vi "Robo Team Send Pitch Rotation Command.vi"(7 "timeout in ms (5000)":i32=5000, 8 "error in (no error)":errorcluster, 10 "Data in":variant, 11 "Command":string) -> (0 "error out":errorcluster, 2 "Data out":variant)   [LabVIEW 2015]
uses:
  Robo Team Engine Command.ctl
  Robo Team Globals.vi
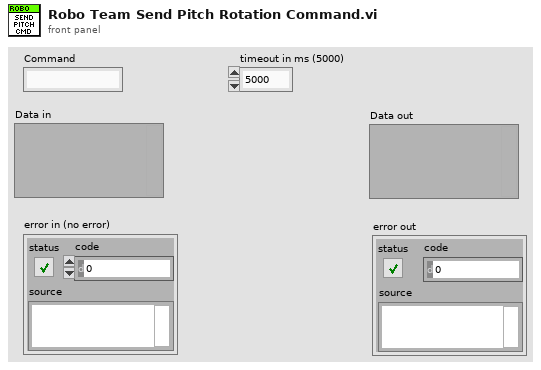
[diagram p1: front panel]
types:
  T1 = typedef "Robo Team Engine Command.ctl" = cluster{"Command":string, "Data":variant, "Error":errorcluster, "Timeout":i32}
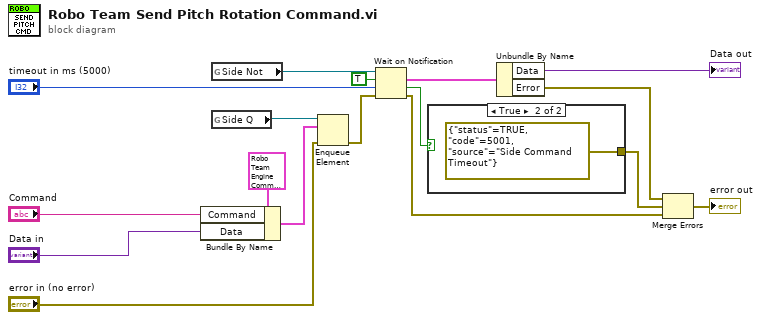
[diagram p0: block diagram]
diagram:
  n1 = Bundle By Name(cluster=T1 {"Command"="", "Data"=variant, "Error"={"status"=FALSE, "code"=0, "source"=""}, "Timeout"=0} ("element"), "Command"="Command", "Data"="Data in") -> (w12:T1)
  n2 = global read "Robo Team Globals.vi" "Side Not"() -> (w8:refnum<notifier>)
  n3 = global read "Robo Team Globals.vi" "Side Q"() -> (w7:refnum<queue>)
  n4 = Enqueue Element(queue=w7, element=w12, error in (no error)="error in (no error)") -> (error out=w9:errorcluster)  [unwired: 1 in, 2 out]
  n5 = Wait on Notification(notifier=w8, ignore previous (F)=TRUE, timeout in ms (-1)="timeout in ms (5000)", error in (no error)=w9) -> (notification=w14:T1, timed out?=w3:bool, error out=w5:errorcluster)  [unwired: 1 out]
  n6 = case shown="True" w3 {
    tunnel: [_ errorcluster {"status"=TRUE, "code"=5001, "source"="Side Command Timeout"} ("Error")] -> w1
    frame False {
    }
    frame True {
    }
  }
  n7 = Unbundle By Name(w14) -> ("Data"=→"Data out":variant, "Error"=w2:errorcluster)
  n8 = Merge Errors(w2, w1, w5) -> (→"error out":errorcluster)
